vi "Write Record.vi"(8 "error in (no error)":errorcluster, 10 "Record":T1 {"Balance" format="%.2f"}, 11 "Configuration Database in":refnum<class "Configuration Database.lvclass">) -> (0 "error out":errorcluster, 3 "Configuration Database out":refnum<class "Configuration Database.lvclass">)   [LabVIEW 2019, in "Configuration Database.lvlib" / "Configuration Database.lvclass"]
uses:
  Configuration Database.lvclass
  Record -Cluster.ctl
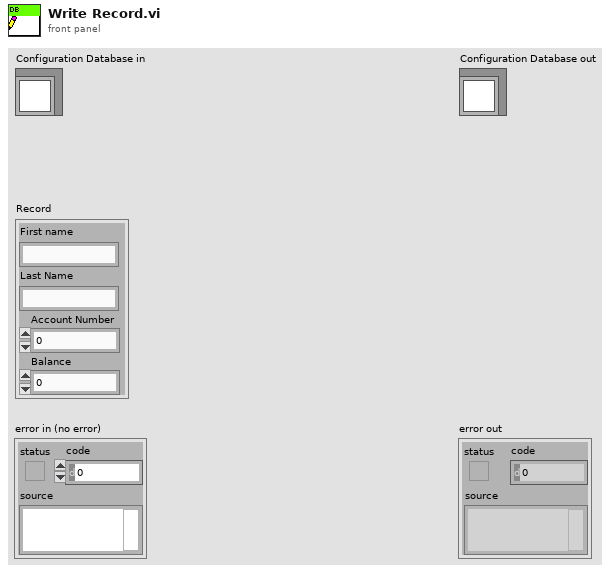
[diagram p1: front panel]
types:
  T1 = typedef "Configuration Database.lvlib/Configuration Database.lvclass/Record -Cluster.ctl" = cluster{"First name":string, "Last Name":string, "Account Number":u16, "Balance":u32}
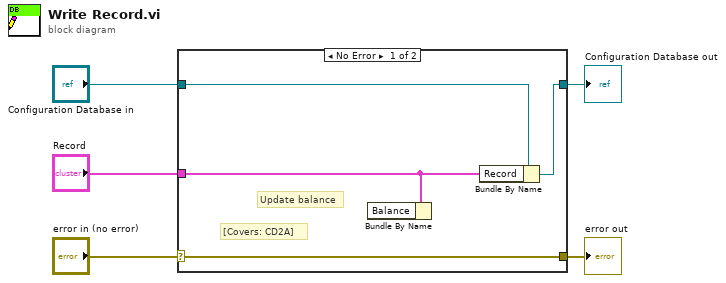
[diagram p0: block diagram]
diagram:
  n1 = case shown="No Error" "error in (no error)" {
    selector: "error in (no error)" -> [w9 w10]
    tunnel: [w9 w10] -> w4
    tunnel: [w7 w11] -> w2
    tunnel: "Configuration Database in" -> [w8 w11]
    tunnel: "Record" -> [w6 _]
    frame No Error {
      # "Update balance"
      # "[Covers: CD2A]"
      n2 = Bundle By Name(cluster=w6) -> ()  [unwired: 1 in, 1 out]
      n3 = Bundle By Name(cluster=w8, "Record"=w6) -> (w7:refnum<class "Configuration Database.lvclass">)
    }
    frame Error {
    }
  }
  "error out" <- w4
  "Configuration Database out" <- w2
